vi "GetContactStatusVI.vi"(8 "error in":errorcluster) -> (0 "error out":errorcluster, 3 "ContactStatusBool":bool)   [LabVIEW 2012]
uses:
  <vilib>/DAQmx/read.llb/DAQmx Read (Digital Bool 1Line 1Point).vi
  <vilib>/DAQmx/miscellaneous.llb/DAQmx Fill In Error Info.vi
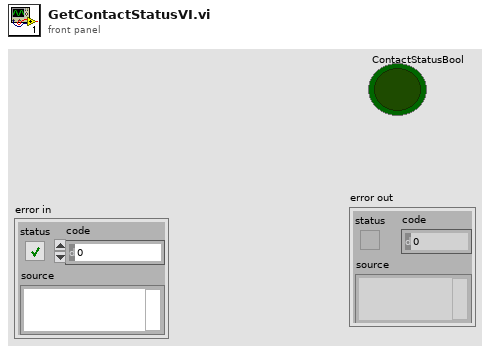
[diagram p1: front panel]
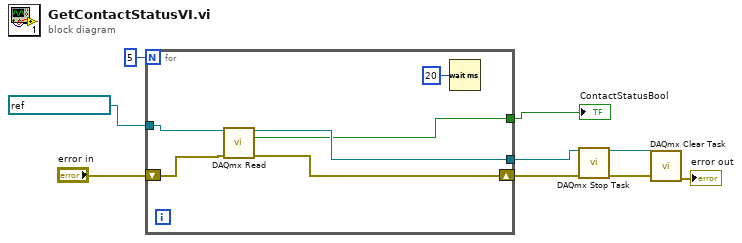
[diagram p0: block diagram]
diagram:
  n1 = for {
    N: 5 -> [_]
    tunnel: refnum<k21> "ContactStatus" -> [w15]
    tunnel: [w13] -> w8
    shift-right: [w12] -> w6
    shift-left: "error in" -> [w11]
    tunnel: [w10] -> w1
    n2 = call-poly <vilib>:"DAQmx Read.vi"("task/channels in"=w15, "error in"=w11) -> ("task out"=w13:refnum<k21>, "data"=w10:bool, "error out"=w12:errorcluster)  [unwired: 11 in]
    n3 = Wait (ms)(milliseconds to wait=u32 20) -> ()  [unwired: 1 out]
  }
  "ContactStatusBool" <- w1
  n4 = call <vilib>:"DAQmx Stop Task.vi"("task/channels in"=w8, "error in"=w6) -> ("task out"=w5:refnum<k21>, "error out"=w4:errorcluster)  [unwired: 12 in]
  n5 = call <vilib>:"DAQmx Clear Task.vi"("task in"=w5, "error in"=w4) -> ("error out"=→"error out":errorcluster)  [unwired: 13 in]
